vi "ESTADO_ACELMTS.vi"(8 "Numeric":i32, 9 "Array 2":bool[](array[boolean]), 10 "Array":bool[](array[boolean])) -> (2 "Array 8":string[](array[string]), 3 "Array 14":string[](array[string]))   [LabVIEW 2015]
panel:
  out "Array 3":string[](array[string])
  out "size(s) 2":i32
  out "size(s)":i32
  out "deleted portion":string
  out "Array 11":i32[](array[numeric])
  out "index of element":i32
  out "array w/ subset deleted":string[](array[string])
  out "Array 12":string[](array[string])
  out "length":i32
  out "Array 7":string[](array[string])
  out "String":string
  out "String 2":string
  out "Array 4":string[](array[string])
  out "appended array":bool[][](array[boolean])
  out "Array 5":string[](array[string])
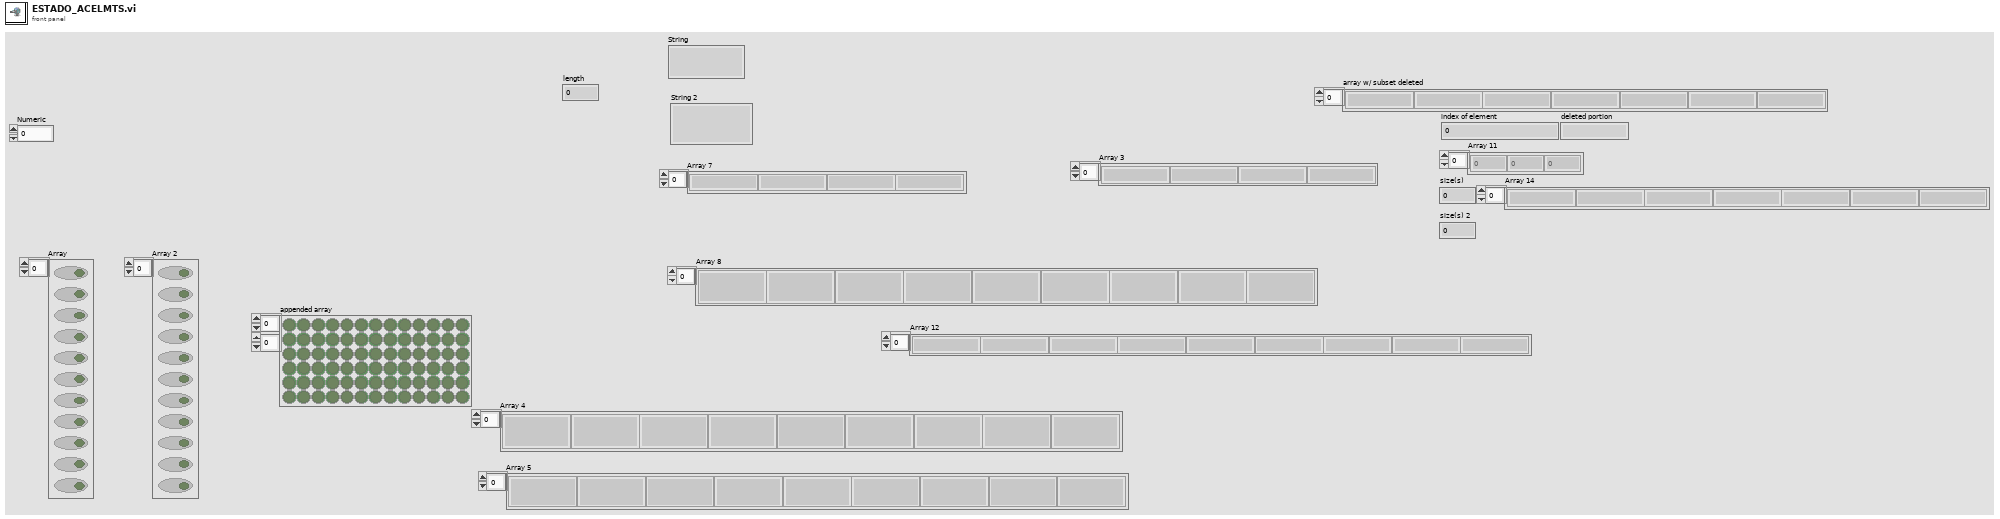
[diagram p1: front panel]
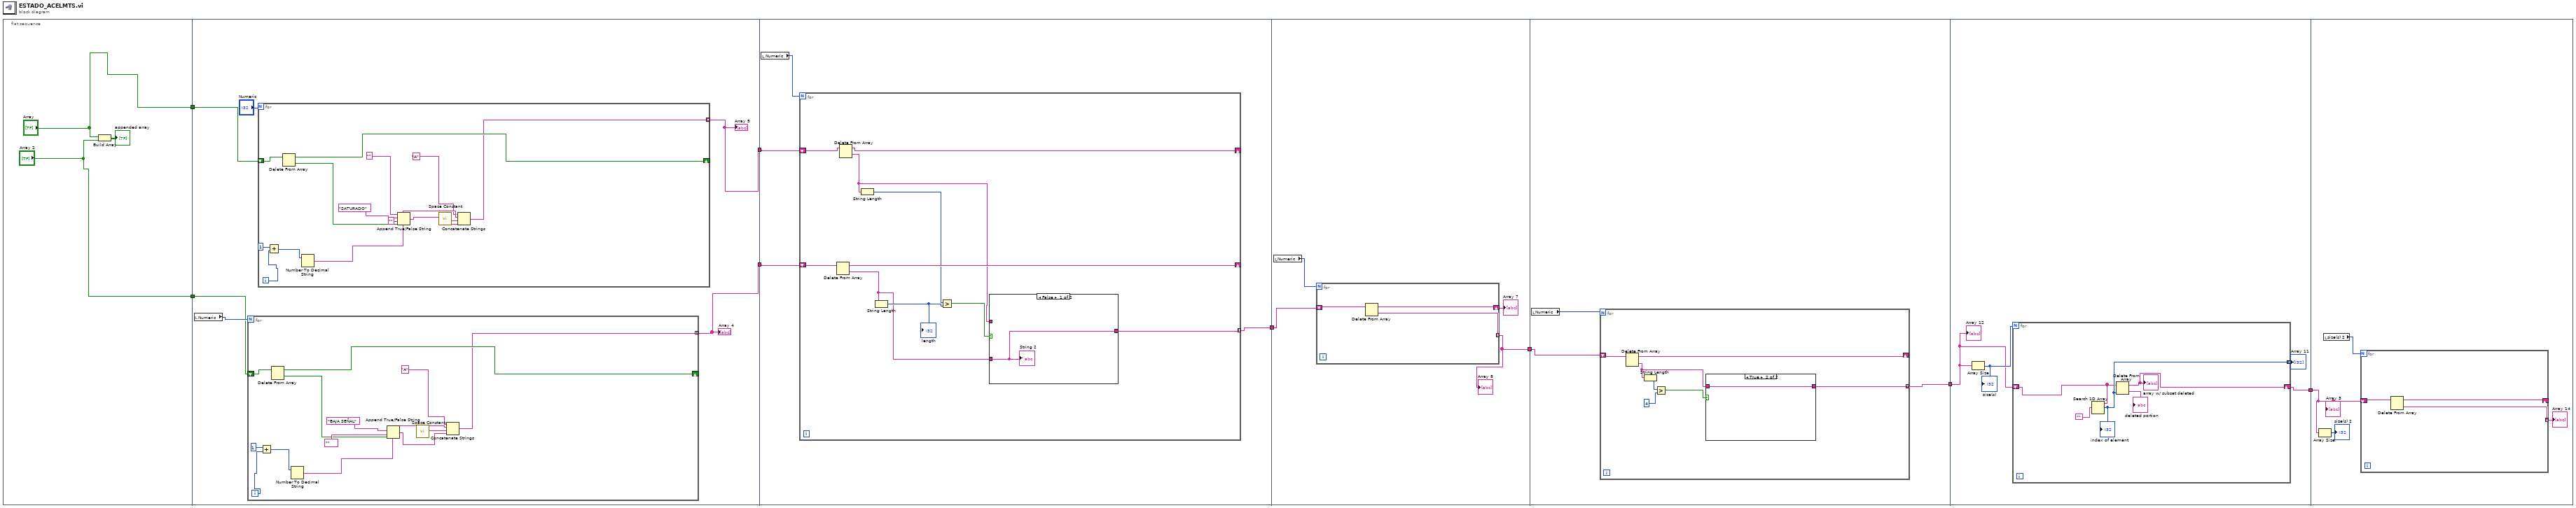
[diagram p0: block diagram]
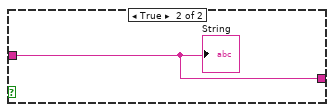
[diagram p2: hidden frame]
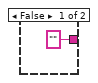
[diagram p3: hidden frame]
diagram:
  n1 = flat-sequence {
    tunnel: ["Array"] -> w8
    tunnel: ["Array 2"] -> w7
    tunnel: w8 -> [w13]
    tunnel: w7 -> [w12]
    tunnel: [w15] -> w6
    tunnel: [w14] -> w5
    tunnel: w6 -> [w47]
    tunnel: w5 -> [w46]
    tunnel: [w45] -> w4
    tunnel: w4 -> [w62]
    tunnel: [w61] -> w3
    tunnel: w3 -> [w69]
    tunnel: [w68] -> w2
    tunnel: w2 -> [w81]
    tunnel: [w80] -> w1
    tunnel: w1 -> [w89]
    frame #0 {
      n2 = Build Array("Array", "Array 2") -> (→"appended array":bool[][])
    }
    frame #1 {
      n3 = local read "Numeric"() -> (w17:i32)
      n4 = for {
        N: w17 -> [_]
        shift-right: [w42] -> _
        shift-left: w12 -> [w43]
        tunnel: [w41] -> w14 mode=indexing
        i -> [w34]
        n5 = Add(x=1, y=w34) -> (x+y=w32:i32)
        n6 = Delete From Array(array=w43) -> (deleted portion=w39:bool, array with subset deleted=w42:bool[])  [unwired: 2 in]
        n7 = Number To Decimal String(number=w32) -> (decimal integer string=w38:string)  [unwired: 1 in]
        n8 = Append True/False String(1:w39, 2:"" ("false string"), 3:"BAJA SEÑAL" ("false string")) -> (0:w36:string)  [unwired: 1 in]
        n9 = call <vilib>:"Space Constant.vi"() -> ("String"=w35:string)
        n10 = Concatenate Strings("A" ("string"), w38, w35, w36) -> (w41:string)
      }
      "Array 4" <- w14
      n11 = for {
        N: "Numeric" -> [_]
        shift-right: [w29] -> _
        shift-left: w13 -> [w30]
        tunnel: [w28] -> w15 mode=indexing
        i -> [w19]
        n12 = Add(x=1, y=w19) -> (x+y=w18:i32)
        n13 = Delete From Array(array=w30) -> (deleted portion=w26:bool, array with subset deleted=w29:bool[])  [unwired: 2 in]
        n14 = Number To Decimal String(number=w18) -> (decimal integer string=w25:string)  [unwired: 1 in]
        n15 = Append True/False String(1:w26, 2:"" ("false string"), 3:"SATURADO" ("false string"), 4:"" ("string (\"\")")) -> (0:w22:string)
        n16 = call <vilib>:"Space Constant.vi"() -> ("String"=w21:string)
        n17 = Concatenate Strings("A" ("string"), w25, w21, w22) -> (w28:string)
      }
      "Array 5" <- w15
    }
    frame #2 {
      n18 = local read "Numeric"() -> (w48:i32)
      n19 = for {
        N: w48 -> [_]
        shift-right: [w57] -> _
        shift-left: w47 -> [w58]
        shift-right: [w55] -> _
        shift-left: w46 -> [w56]
        tunnel: [w49] -> w45 mode=indexing
        n20 = Delete From Array(array=w56) -> (deleted portion=w50:string, array with subset deleted=w55:string[])  [unwired: 2 in]
        n21 = Delete From Array(array=w58) -> (deleted portion=w51:string, array with subset deleted=w57:string[])  [unwired: 2 in]
        n22 = String Length(string=w51) -> (length=w54:i32)
        n23 = String Length(string=w50) -> (length=w53:i32)
        "length" <- w53
        n24 = Greater?(x=w54, y=w53) -> (0:w52:bool)
        n25 = case shown="False" w52 {
          tunnel: w51 -> [_ w60]
          tunnel: w50 -> [w59 _]
          tunnel: [w59 w60] -> w49
          frame False {
            "String 2" <- w59
          }
          frame True {
            "String" <- w60
          }
        }
      }
    }
    frame #3 {
      n26 = local read "Numeric"() -> (w63:i32)
      n27 = for {
        N: w63 -> [_]
        shift-right: [w66] -> w64
        shift-left: w62 -> [w67]
        tunnel: [w65] -> w61 mode=indexing
        n28 = Delete From Array(array=w67) -> (deleted portion=w65:string, array with subset deleted=w66:string[])  [unwired: 2 in]
      }
      "Array 7" <- w64
      "Array 8" <- w61
    }
    frame #4 {
      n29 = local read "Numeric"() -> (w70:i32)
      n30 = for {
        N: w70 -> [_]
        shift-right: [w76] -> _
        shift-left: w69 -> [w77]
        tunnel: [w71] -> w68 mode=indexing
        n31 = Delete From Array(array=w77) -> (deleted portion=w72:string, array with subset deleted=w76:string[])  [unwired: 2 in]
        n32 = String Length(string=w72) -> (length=w75:i32)
        n33 = Greater?(x=w75, y=4) -> (0:w73:bool)
        n34 = case shown="True" w73 {
          tunnel: w72 -> [_ w79]
          tunnel: ["" w79] -> w71
          frame False {
          }
          frame True {
          }
        }
      }
    }
    frame #5 {
      n35 = Array Size(array=w81) -> (size(s)=w82:i32)
      "size(s)" <- w82
      n36 = for {
        N: w82 -> [_]
        tunnel: [w87] -> w83 mode=indexing
        shift-right: [w84] -> w80
        shift-left: w81 -> [w85]
        n37 = Search 1D Array(1D array=w85, element="") -> (index of element=w87:i32)  [unwired: 1 in]
        "index of element" <- w87
        n38 = Delete From Array(array=w85, index=w87) -> (deleted portion=→"deleted portion":string, array with subset deleted=w84:string[])  [unwired: 1 in]
        "array w/ subset deleted" <- w84
      }
      "Array 11" <- w83
      "Array 12" <- w81
    }
    frame #6 {
      n39 = Array Size(array=w89) -> (size(s)=→"size(s) 2":i32)
      n40 = local read "size(s) 2"() -> (w92:i32)
      n41 = for {
        N: w92 -> [_]
        shift-right: [w94] -> _
        shift-left: w89 -> [w95]
        tunnel: [w93] -> w90 mode=indexing
        n42 = Delete From Array(array=w95) -> (deleted portion=w93:string, array with subset deleted=w94:string[])  [unwired: 2 in]
      }
      "Array 14" <- w90
      "Array 3" <- w89
    }
  }
